vi "SetStatus.vi"(4 "Append timestamp?":bool, 6 "Label":string, 9 "Error?":bool, 10 "Description":string, 11 "Code":i32) -> (1 "Error out":errorcluster)   [LabVIEW 2017, in "GPError.lvlib"]
doc: "Sets an error or warning (depending on <B>Error?</B>) on <B>Error out</B> specified by <B>Code</B>, <B>Label</B>, and <B>Description</B>.\n\nThe call chain will always be set in <B>Error out</B> source, and description(s) will be appended from one or more of these sources (in the following order):\n\n1) If any built-in or user defined error/warning descriptions exist in LabVIEW's database these will come first.\n\n2) If any custom descriptions are defined for <B>Code</B> (with the DefineCustomCode function), these will be appended to the built-in descriptions. If no built-in descriptions exist the custom descriptions are used by themselves.\n\n3) If anything but an empty string is wired to the <B>Description</B> input this will be appended to any of the above or used by itself if nothing else is defined. This lets you add a final qualifier or give additional info to the specific error on top of the pre-defined, and maybe somewhat generic, descriptions (e.g. \"This error was caused by this specific module not loading due to timeout of X seconds\").\n\n<B>Append timestamp?</B> specifies if the current UTC time and date will be appended to the source string.\n\nSteen Schmidt\nGPower\n10/7 2013"
uses:
  GPError.lvlib
  FG/CustomErrorFGFunction.ctl
panel:
  # "Copyright © 2013\nSteen Schmidt, GPower\nSee enclosed license file for terms and conditions"
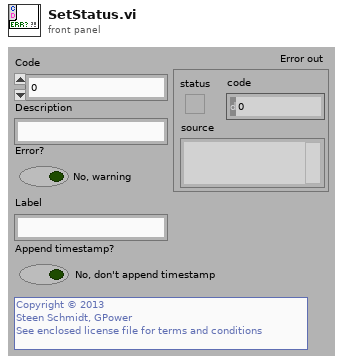
[diagram p1: front panel]
types:
  T1 = typedef "GPError.lvlib/CustomErrorFGFunction.ctl" = enum16{"Get custom descriptions", "Set custom code", "Unset custom code"}
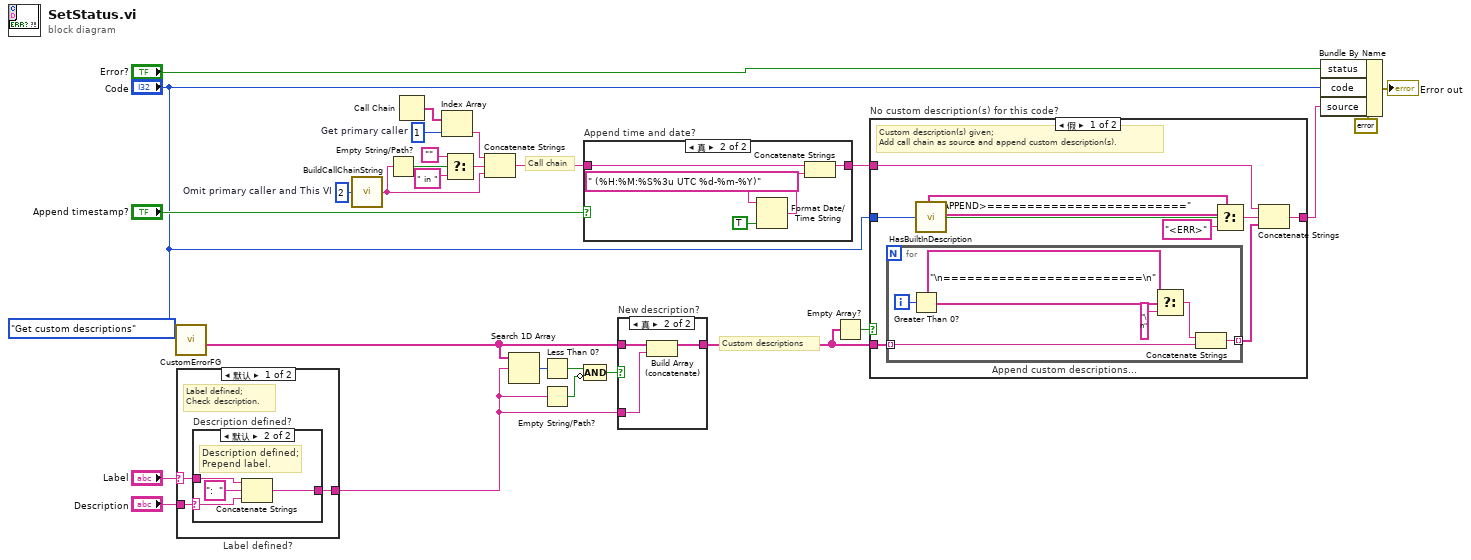
[diagram p0: block diagram]
diagram:
  w15 = 2  # Omit primary caller and This VI
  w13 = 1  # Get primary caller
  # "Call chain"
  # "Custom descriptions"
  n1 = call "CustomErrorFG.vi"("Custom code"="Code", "Function"=CustomErrorFGFunction."Get custom descriptions") -> ("Custom descriptions out"=w23:string[])  [unwired: 8 in, 1 out]
  n2 = case "Label defined?" shown="默认" "Label" {
    selector: "Label" -> [w31 _]
    tunnel: "Description" -> [w29 w36]
    tunnel: [w30 w36] -> w1
    frame Default {
      # "Label defined;\nCheck description."
      n3 = case "Description defined?" shown="默认" w29 {
        selector: w29 -> [_ w32]
        tunnel: w31 -> [_ w35]
        tunnel: [_ w33] -> w30
        frame "" {
          # "No description defined;\nOmit label as well."
        }
        frame Default {
          # "Description defined;\nPrepend label."
          n4 = Concatenate Strings(w35, ":  ", w32) -> (w33:string)
        }
      }
    }
    frame "" {
      # "No label defined;\nJust use description."
    }
  }
  n5 = call "BuildCallChainString.vi"("Lower levels to omit"=w15) -> ("Call chain string"=w20:string)  [unwired: 4 in]
  n6 = Empty String/Path?(string/path=w20) -> (empty?=w16:bool)
  n7 = Call Chain() -> (call chain=w12:string[])
  n8 = Index Array(array=w12, index=w13) -> (element=w14:string)
  n9 = Select(t="", s=w16, f=" in ") -> (s? t:f=w19:string)
  n10 = Concatenate Strings(w14, w19, w20) -> (w7:string)
  n11 = Search 1D Array(1D array=w23, element=w1) -> (index of element=w9:i32)  [unwired: 1 in]
  n12 = Less Than 0?(x=w9) -> (x < 0?=w11:bool)
  n13 = Empty String/Path?(string/path=w1) -> (empty?=w10:bool)
  n14 = case "Append time and date?" shown="真" "Append timestamp?" {
    tunnel: w7 -> [w37 w40]
    tunnel: [w37 w38] -> w5
    frame False {
    }
    frame True {
      n15 = Format Date/Time String(time format string (%c)=" (%H:%M:%S%3u UTC %d-%m-%Y)", UTC format=TRUE) -> (date/time string=w39:string)  [unwired: 1 in]
      n16 = Concatenate Strings(w40, w39) -> (w38:string)
    }
  }
  n17 = Compound Arithmetic op=AND(w11, invert w10) -> (w8:bool)
  n18 = case "New description?" shown="真" w8 {
    tunnel: w23 -> [w43 w46]
    tunnel: [w43 w44] -> w22
    tunnel: w1 -> [_ w45]
    frame False {
    }
    frame True {
      n19 = Build Array (concatenate)(w46, w45) -> (w44:string[])
    }
  }
  n20 = Empty Array?(array=w22) -> (empty?=w21:bool)
  n21 = case "No custom description(s) for this code?" shown="假" w21 {
    tunnel: w22 -> [w49 _]
    tunnel: [w55 w63] -> w27
    tunnel: "Code" -> [w54 _]
    tunnel: w5 -> [w47 w63]
    frame False {
      # "Custom description(s) given;\nAdd call chain as source and append custom description(s)."
      n22 = for "Append custom descriptions..." {
        tunnel: w49 -> [w62] mode=indexing
        tunnel: [w57] -> w48 mode=indexing
        i -> [w61]
        n23 = Greater Than 0?(x=w61) -> (x > 0?=w60:bool)
        n24 = Select(t="\n=========================\n", s=w60, f="\n") -> (s? t:f=w59:string)
        n25 = Concatenate Strings(w59, w62) -> (w57:string)
      }
      n26 = call "HasBuiltInDescription.vi"("Error/warning code"=w54) -> ("Has built-in description?"=w53:bool)  [unwired: 4 in]
      n27 = Select(t="<APPEND>=========================", s=w53, f="<ERR>") -> (s? t:f=w51:string)
      n28 = Concatenate Strings(w47, w51, w48) -> (w55:string)
    }
    frame True {
      # "No custom descriptions;\nJust add call chain as source."
    }
  }
  n29 = Bundle By Name(cluster=errorcluster {"status"=FALSE, "code"=0, "source"=""} ("error out"), "status"="Error?", "code"="Code", "source"=w27) -> (→"Error out":errorcluster)
